vi "GetWorldPosition.vi"(8 "group":i32, 10 "Snpx":refnum<k24>, 11 "error in":errorcluster) -> (0 "UserTool":i16, 1 "Cartesian position":T1, 2 "JointsPosition":dbl[](array[numeric]), 3 "error out":errorcluster)   [LabVIEW 2010, in "UnderAutomation.Fanuc.lvlib"]
uses:
  UnderAutomation.Fanuc.lvlib
  C:/Users/fg/Documents/Fanuc.vi/LabVIEW_2024/UnderAutomation.Fanuc/lib/UnderAutomation.Fanuc.dll
  LabVIEW_2024/UnderAutomation.Fanuc/lib/UnderAutomation.Fanuc.dll
panel:
  out "UserFrame":i16
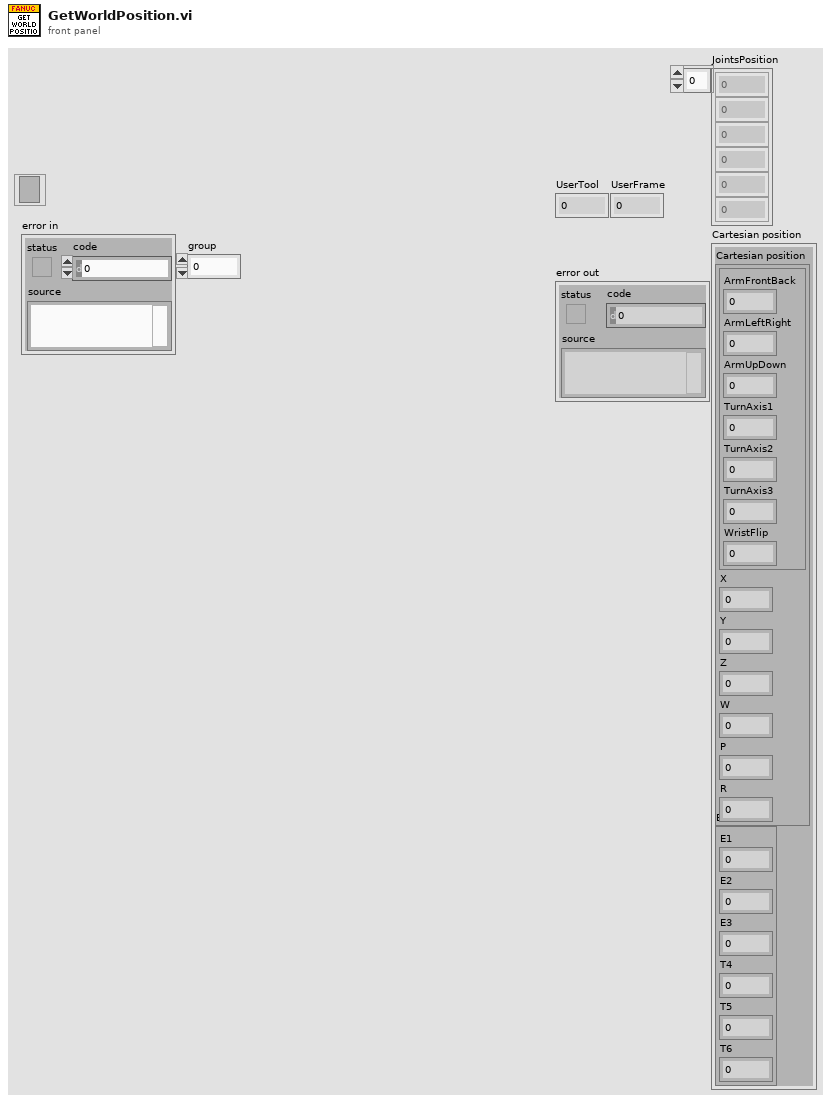
[diagram p1: front panel]
types:
  T1 = cluster{"Cartesian position":cluster{cluster{"ArmFrontBack":i32, "ArmLeftRight":i32, "ArmUpDown":i32, "TurnAxis1":i32, "TurnAxis2":i32, "TurnAxis3":i32, "WristFlip":i32}, "X":dbl, "Y":dbl, "Z":dbl, "W":dbl, "P":dbl, "R":dbl}, "Extension":cluster{"E1":dbl, "E2":dbl, "E3":dbl, "T4":i16, "T5":i16, "T6":i16}}
  T2 = cluster{"Configuration":cluster{"ArmFrontBack":i32, "ArmLeftRight":i32, "ArmUpDown":i32, "TurnAxis1":i32, "TurnAxis2":i32, "TurnAxis3":i32, "WristFlip":i32}, "X":dbl, "Y":dbl, "Z":dbl, "W":dbl, "P":dbl, "R":dbl}
  T3 = cluster{"E1":dbl, "E2":dbl, "E3":dbl, "T4":i16, "T5":i16, "T6":i16}
  T4 = cluster{"Cartesian position":cluster{"Configuration":cluster{"ArmFrontBack":i32, "ArmLeftRight":i32, "ArmUpDown":i32, "TurnAxis1":i32, "TurnAxis2":i32, "TurnAxis3":i32, "WristFlip":i32}, "X":dbl, "Y":dbl, "Z":dbl, "W":dbl, "P":dbl, "R":dbl}, cluster{"E1":dbl, "E2":dbl, "E3":dbl, "T4":i16, "T5":i16, "T6":i16}}
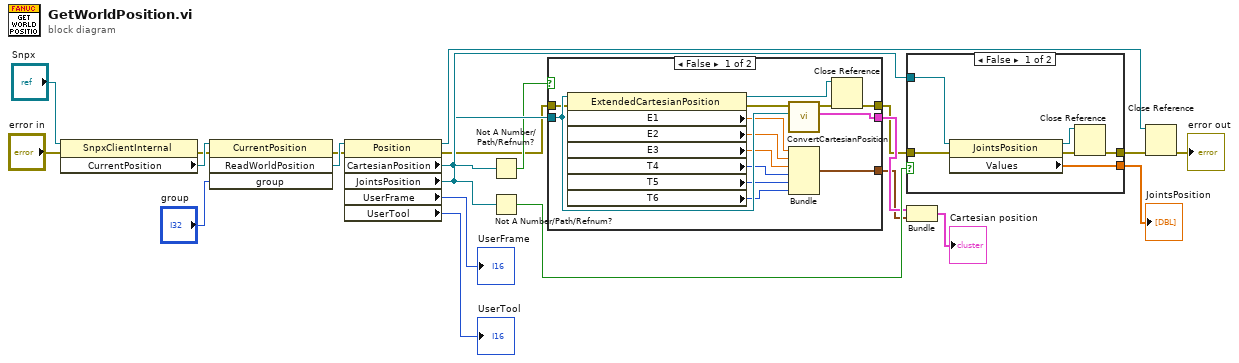
[diagram p0: block diagram]
diagram:
  n1 = property class="SnpxClientInternal"(reference="Snpx", error in="error in") -> (error out=w19:errorcluster, "CurrentPosition"=w20:refnum<k24>)  [unwired: 1 out]
  n2 = invoke class="CurrentPosition" method="ReadWorldPosition"(reference=w20, error in=w19, "group"="group") -> (error out=w3:errorcluster, "ReadWorldPosition"=w18:refnum<k24>)  [unwired: 1 in, 2 out]
  n3 = property class="Position"(reference=w18, error in=w3) -> (reference out=w17:refnum<k24>, error out=w6:errorcluster, "CartesianPosition"=w11:refnum<k24>, "JointsPosition"=w13:refnum<k24>, "UserFrame"=→"UserFrame":i16, "UserTool"=→"UserTool":i16)
  n4 = Not A Number/Path/Refnum?(number/path/refnum=w11) -> (NaN/Path/Refnum?=w10:bool)
  n5 = Not A Number/Path/Refnum?(number/path/refnum=w13) -> (NaN/Path/Refnum?=w14:bool)
  n6 = case shown="False" w10 {
    tunnel: w11 -> [w35 _]
    tunnel: [w36 _] -> w9
    tunnel: [w28 _] -> w8
    tunnel: w6 -> [w27 w37]
    tunnel: [w25 w37] -> w5
    frame False {
      n7 = property class="ExtendedCartesianPosition"(reference=w35, error in=w27) -> (reference out=w26:refnum<k24>, error out=w24:errorcluster, "E1"=w34:dbl, "E2"=w33:dbl, "E3"=w32:dbl, "T4"=w31:i16, "T5"=w30:i16, "T6"=w29:i16)
      n8 = call "ConvertCartesianPosition.vi"("Cartesian position"=w35, "error in (no error)"=w24) -> ("Cartesian position"=w36:T2, "error out"=w23:errorcluster)  [unwired: 8 in]
      n9 = Bundle("E1"=w34, "E2"=w33, "E3"=w32, "T4"=w31, "T5"=w30, "T6"=w29) -> (w28:T3)  [unwired: 1 in]
      n10 = Close Reference(reference=w26, error in (no error)=w23) -> (error out=w25:errorcluster)
    }
    frame True {
    }
  }
  n11 = case shown="False" w14 {
    tunnel: w13 -> [w43 _]
    tunnel: [w42 _] -> w12
    tunnel: w5 -> [w39 w44]
    tunnel: [w38 w44] -> w4
    frame False {
      n12 = property class="JointsPosition"(reference=w43, error in=w39) -> (reference out=w40:refnum<k24>, error out=w41:errorcluster, "Values"=w42:dbl[])
      n13 = Close Reference(reference=w40, error in (no error)=w41) -> (error out=w38:errorcluster)
    }
    frame True {
    }
  }
  "JointsPosition" <- w12
  n14 = Bundle("Cartesian position"=w9, w8) -> (→"Cartesian position":T4)  [unwired: 1 in]
  n15 = Close Reference(reference=w17, error in (no error)=w4) -> (error out=→"error out":errorcluster)
